vi "Wait Test.vi"() -> ()   [LabVIEW 2024]
uses:
  Shared/Steps/Shared Steps.lvlib
panel:
  out "Duration (ms)":u32
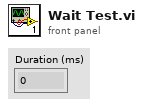
[diagram p1: front panel]
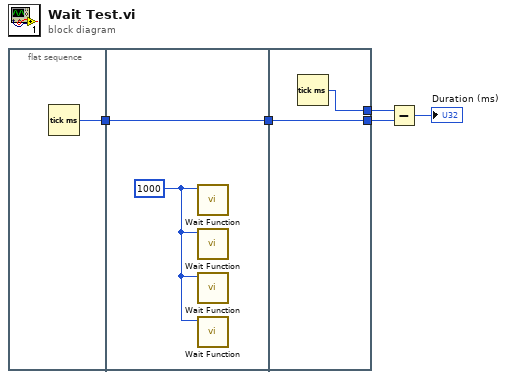
[diagram p0: block diagram]
diagram:
  n1 = flat-sequence {
    tunnel: [w6] -> w4
    tunnel: w4 -> [w7]
    tunnel: [w7] -> w3
    tunnel: [w10] -> w5
    tunnel: w3 -> [w9]
    tunnel: [w9] -> w2
    frame #0 {
      n2 = Tick Count (ms)() -> (millisecond timer value=w6:u32)
    }
    frame #1 {
      w8 = u32 1000 ("Wait (ms)")
      n3 = call "Wait Function.vi"("Wait (ms)"=w8) -> ()  [unwired: 10 in, 1 out]
      n4 = call "Wait Function.vi"("Wait (ms)"=w8) -> ()  [unwired: 10 in, 1 out]
      n5 = call "Wait Function.vi"("Wait (ms)"=w8) -> ()  [unwired: 10 in, 1 out]
      n6 = call "Wait Function.vi"("Wait (ms)"=w8) -> ()  [unwired: 10 in, 1 out]
    }
    frame #2 {
      n7 = Tick Count (ms)() -> (millisecond timer value=w10:u32)
    }
  }
  n8 = Subtract(x=w5, y=w2) -> (x-y=→"Duration (ms)":u32)
